vi "macro_PosCtrl_Execute.vi"() -> ()   [LabVIEW 2019, in "Trajectory_Library.lvlib"]
uses:
  Trajectory_Library.lvlib
panel:
  in  "CurrentPosition":dbl
  in  "TargetPosition":dbl
  out "Output":dbl
  out "OnTarget":bool
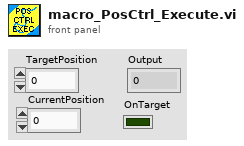
[diagram p1: front panel]
types:
  T1 = typedef "Trajectory_Library.lvlib/PosCtrl_Tuning_Type.ctl" = cluster{"Slope":dbl, "Offset":dbl, "Error Deadband":dbl, "At Reference Count":i32, "Negate Output":bool, "Max Allowd Position":dbl, "Min Allowd Position":dbl}
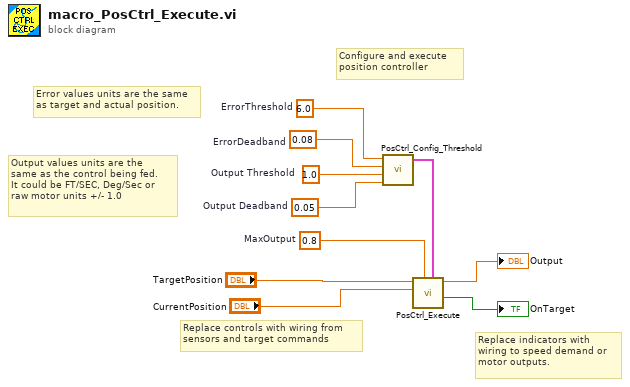
[diagram p0: block diagram]
diagram:
  w1 = 0.8  # MaxOutput
  w7 = 6.0  # ErrorThreshold
  w8 = 0.08  # ErrorDeadband
  w9 = 1.0  # Output Threshold
  w10 = 0.05  # Output Deadband
  # "Replace controls with wiring from\nsensors and target commands"
  # "Replace indicators with\nwiring to speed demand or\nmotor outputs."
  # "Output values units are the\nsame as the control being fed.  \nIt could be FT/SEC, Deg/Sec or\nraw motor units +/- 1.0"
  # "Error values units are the same \nas target and actual position."
  # "Configure and execute \nposition controller"
  n1 = call "PosCtrl_Config_Threshold.vi"("Output Deadband"=w10, "Output Threshold"=w9, "ErrorDeadband"=w8, "ErrorThreshold"=w7) -> ("PosCtrl_Config_Params"=w6:T1)  [unwired: 7 in]
  n2 = call "PosCtrl_Execute.vi"("PosCtrl_Config_Params"=w6, "MaxOutput"=w1, "CurrentPosition"="CurrentPosition", "TargetPosition"="TargetPosition") -> ("OnTarget"=→"OnTarget":bool, "Output"=→"Output":dbl)  [unwired: 5 in, 1 out]
